vi "_convert_response_to_float_scalar_number.vi"(8 "error in":errorcluster caption="error in (no error)", 10 "Input string":string, 11 "VISA resource name":refnum<visa-resource-name>) -> (0 "error out":errorcluster, 2 "Double out":dbl format="%#_p", 3 "VISA resource name out":refnum<visa-resource-name>)   [LabVIEW 2020, in "Rohde&Schwarz RTx Oscilloscopes.lvlib" / "rsidr_core.lvlib"]
doc: "Queries array of floats that can be returned in ASCII format or in binary format. The array is always returned as the most-universal double array.\n- For <b>ASCII</b> format, the array numbers are decoded as comma-separated values.\n- For <b>Binary Format</b>, the numbers are decoded based on the session parameter <b>Bin Float Number Format</b>, usually float 32-bit (REAL,32), swapped endianess (instruments usually use low endian, LabVIEW uses big endian)."
uses:
  rsidr_core.lvlib
  type_AdditionalFlag_Bits.ctl
  type_Error_Codes.ctl
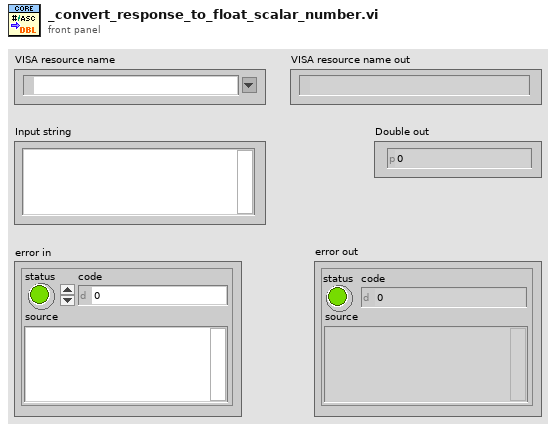
[diagram p1: front panel]
types:
  T1 = typedef "Rohde&Schwarz RTx Oscilloscopes.lvlib/rsidr_core.lvlib/type_AdditionalFlag_Bits.ctl" = enum16{"Send LF after Bin Block", "Junk read with io_clear_buffers.vi", "io_clear_buffers: viClear()", "io_clear_buffers: viFlush()", "<NotUsed1>", "Allow Dbl & Int Bin/Ascii read", "*OPC? in check_instrument_error.vi", "<NotUsed2>", "Smart Enum Matching", "Less Strict RepCaps check", "AssureResponseEndWithLF"}
  T2 = typedef "Rohde&Schwarz RTx Oscilloscopes.lvlib/rsidr_core.lvlib/type_Error_Codes.ctl" = enum16{"No_error", "VISA_err_ResourceNotFound", "VISA_err_Timeout", "VISA_warn_MoreDataAvailable", "RS_err_MissingCallback", "RS_err_InvalidAttribute", "RS_err_InvalidValue", "RS_err_UnknownResource", "RS_err_AlreadyInitialized", "RS_err_InstrumentStatus", "RS_err_BadRepCapName", "RS_err_TypesMismatch", "RS_err_ValueNotSupported", "RS_err_InvalidRngTable", "RS_err_IDqueryFail", "RS_err_UnexpResponse", "VISA_warn_ConfigNotLoaded", "RS_err_AttributeNotReadable", "RS_err_AttributeNotWritable", "RS_err_InstrumentType", "RS_err_InstrumentOption", "VISA_err_InvalidSize", "RS_err_ReliabilityIndicator", "VISA_warn_UnknownStatus", "VISA_warn_TermCharRead", "VISA_err_IO_error", "RS_err_FunctionNotSupported", "VISA_warn_QueueEmpty"}
  T3 = typedef "Rohde&Schwarz RTx Oscilloscopes.lvlib/rsidr_core.lvlib/type_Session_Data.ctl" = cluster{"IDN string":string, "Instrument FW":string, "Instr type":string, "Instr type for err. msg.":string, "Installed Options":string[], "Ignore Error Messages":string, "Logging params":variant, "OPC Timeout":i32, "VISA Timeout":i32, "STB Poll VISA Timeout":i32, "Additional Flags":i32, "Wait Before Read":i32, "Wait Before Write":i32, "Option String Flags":i32, "IO Segment Size":i64, "VISA Access Mode":T4, "Interface Type":T5, "OPC Wait Mode":T6, "Bin Float Number  Format":T7, "Bin Integer Number Format":T8, "Simulate":bool, "VXIcapable":bool, "Duplicate Session":bool, "Add LF to Write":bool, "Logging":bool, "Fast Sweep":bool, "Query Instrument Status":bool, "Check Range":bool, "Check Options":bool, "OPC-sync Attr Writes":bool, "OPC-sync Attr Queries":bool}
  T4 = typedef "Rohde&Schwarz RTx Oscilloscopes.lvlib/rsidr_core.lvlib/type_VisaAccessMode.ctl" = u16
  T5 = typedef "Rohde&Schwarz RTx Oscilloscopes.lvlib/rsidr_core.lvlib/type_InterfaceType.ctl" = enum16{"Unknown", "GPIB", "VXI", "GPIB_VXI", "ASRL", "PXI", "TCPIP", "USB", "SOCKET"}
  T6 = typedef "Rohde&Schwarz RTx Oscilloscopes.lvlib/rsidr_core.lvlib/type_OPC_Wait_Mode.ctl" = enum16{"STBpolling", "STBpollingSlow", "STBpollingSuperSlow", "ServiceRequest", "OPCquery"}
  T7 = typedef "Rohde&Schwarz RTx Oscilloscopes.lvlib/rsidr_core.lvlib/type_Binary_Float_Number_Format.ctl" = enum16{"Float_4_Bytes_Swapped", "Float_4_Bytes", "Double_8_Bytes_Swapped", "Double_8_Bytes"}
  T8 = typedef "Rohde&Schwarz RTx Oscilloscopes.lvlib/rsidr_core.lvlib/type_Binary_Integer_Number_Format.ctl" = enum16{"Int32_4_Bytes_Swapped", "Int32_4 Bytes", "Int16_2_Bytes_Swapped", "Int16_2_Bytes"}
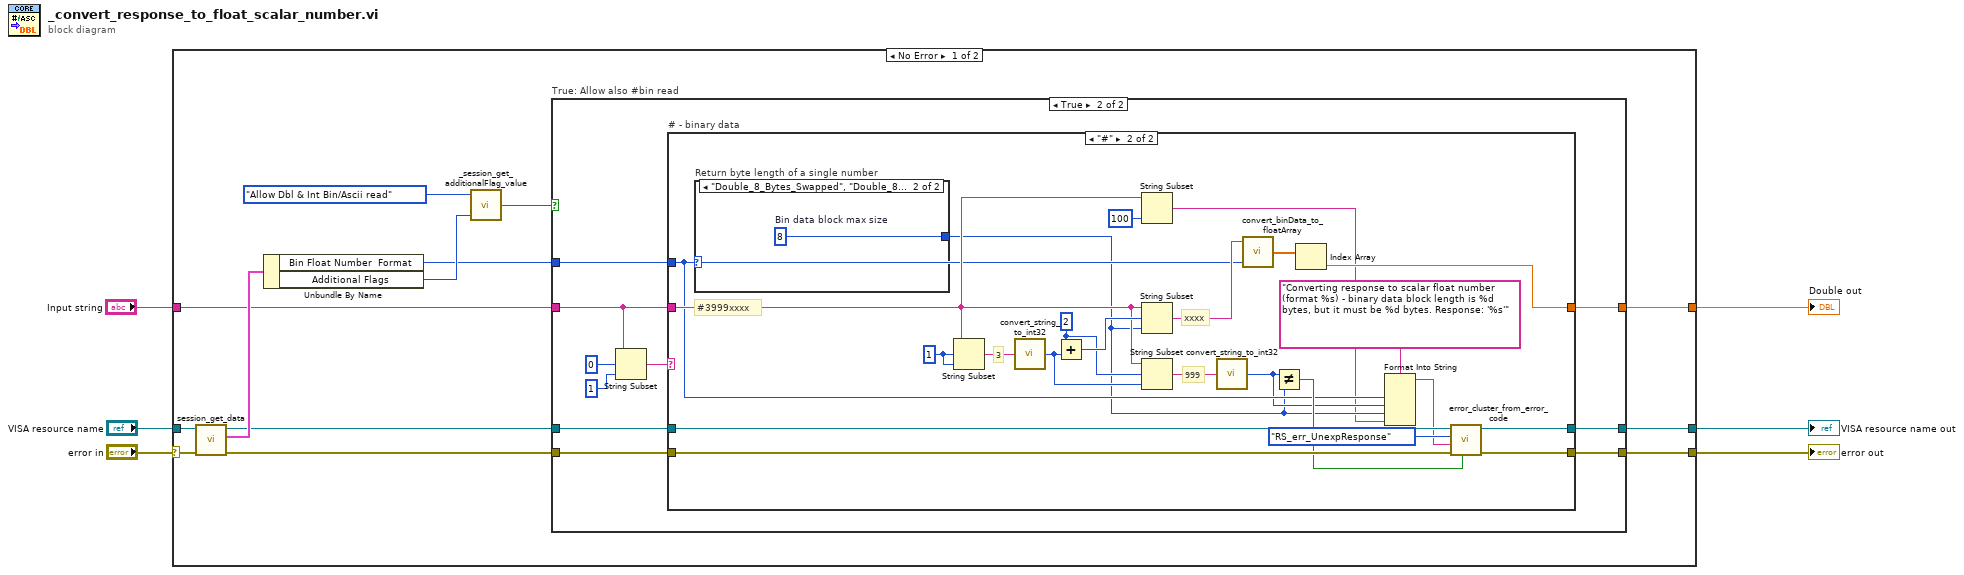
[diagram p0: block diagram]
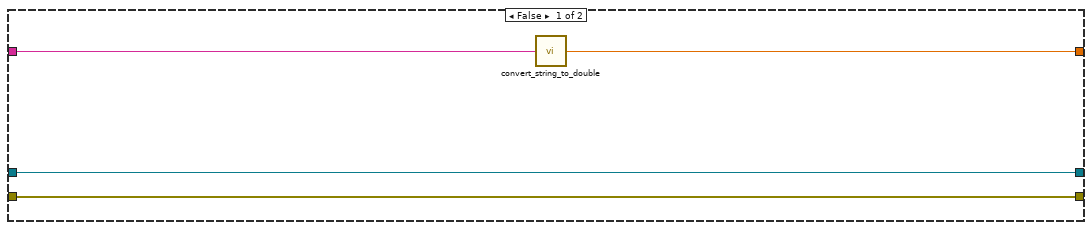
[diagram p2: hidden frame]
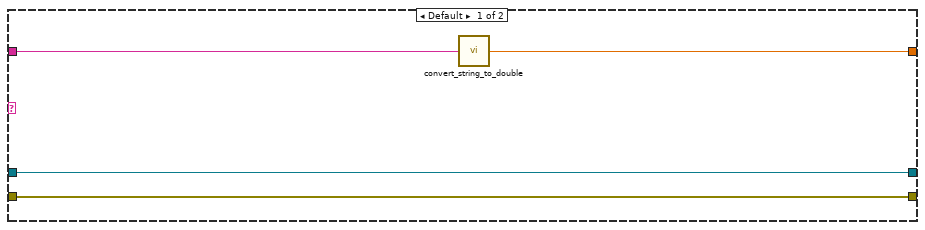
[diagram p3: hidden frame]
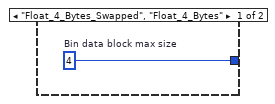
[diagram p4: hidden frame]
diagram:
  n1 = case shown="No Error" "error in" {
    selector: "error in" -> [w19 w64]
    tunnel: [w7 w63] -> w3
    tunnel: [w8 w64] -> w4
    tunnel: "VISA resource name" -> [w18 w63]
    tunnel: [w12 _] -> w1
    tunnel: "Input string" -> [w11 _]
    frame No Error {
      n2 = call "session_get_data.vi"("error in"=w19, "VISA resource name"=w18) -> ("error out"=w10:errorcluster, "Session User Data out"=w17:T3, "VISA resource name out"=w9:refnum<visa-resource-name>)  [unwired: 6 in, 1 out]
      n3 = Unbundle By Name(w17) -> ("Bin Float Number  Format"=w14:T7, "Additional Flags"=w15:i32)
      n4 = call "_session_get_additionalFlag_value.vi"("AdditionalFlags value in"=w15, "AdditionalFlag bit"=type_AdditionalFlag_Bits."Allow Dbl & Int Bin/Ascii read") -> ("AdditionalFlag bit value out"=w13:bool)  [unwired: 3 in]
      n5 = case "True: Allow also #bin read" shown="True" w13 {
        tunnel: w14 -> [_ w25]
        tunnel: [w22 w27] -> w12
        tunnel: w11 -> [w23 w26]
        tunnel: w10 -> [w21 w30]
        tunnel: w9 -> [w20 w31]
        tunnel: [w21 w28] -> w8
        tunnel: [w20 w29] -> w7
        frame False {
          n6 = call "convert_string_to_double.vi"("String in"=w23) -> ("double value out"=w22:dbl)  [unwired: 4 in]
        }
        frame True {
          n7 = String Subset(string=w26, offset (0)=0, length (rest)=1 ("length (rest)")) -> (substring=w24:string)
          n8 = case "# - binary data" shown="\"#\"" w24 {
            tunnel: w26 -> [w37 w43]
            tunnel: w25 -> [_ w41]
            tunnel: [w36 w56] -> w27
            tunnel: w30 -> [w35 w50]
            tunnel: w31 -> [w34 w49]
            tunnel: [w35 w48] -> w28
            tunnel: [w34 w47] -> w29
            frame Default {
              n9 = call "convert_string_to_double.vi"("String in"=w37) -> ("double value out"=w36:dbl)  [unwired: 4 in]
            }
            frame "#" {
              w54 = 2 ("offset (0)")
              w60 = 1 ("offset (0)")
              # "xxxx"
              # "999"
              # "3"
              # "#3999xxxx"
              n10 = case "Return byte length of a single number" shown="\"Double_8_Bytes_Swapped\", \"Double_8_Bytes\"" w41 {
                tunnel: [w61 w62] -> w39
                frame "Float_4_Bytes_Swapped", "Float_4_Bytes" {
                  w61 = 4  # Bin data block max size
                }
                frame "Double_8_Bytes_Swapped", "Double_8_Bytes" {
                  w62 = 8  # Bin data block max size
                }
              }
              n11 = String Subset(string=w43, offset (0)=w60, length (rest)=w60) -> (substring=w59:string)
              n12 = call "convert_string_to_int32.vi"("String in"=w59) -> ("int32 value out"=w53:i32)  [unwired: 4 in]
              n13 = Add(x=w54, y=w53) -> (x+y=w55:i32)
              n14 = String Subset(string=w43, length (rest)=100 ("length (rest)")) -> (substring=w38:string)  [unwired: 1 in]
              n15 = String Subset(string=w43, offset (0)=w55, length (rest)=w39) -> (substring=w58:string)
              n16 = String Subset(string=w43, offset (0)=w54, length (rest)=w53) -> (substring=w52:string)
              n17 = call "convert_string_to_int32.vi"("String in"=w52) -> ("int32 value out"=w40:i32)  [unwired: 4 in]
              n18 = call "convert_binData_to_floatArray.vi"("Bin Float Number Format"=w41, "Bin Data"=w58) -> ("Numbers out"=w57:dbl[])  [unwired: 1 in, 2 out]
              n19 = Not Equal?(x=w40, y=w39) -> (x != y?=w46:bool)
              n20 = Index Array(array=w57) -> (element=w56:dbl)  [unwired: 1 in]
              n21 = Format Into String(format string="Converting response to scalar float number (format %s) - binary data block length is %d bytes, but it must be %d bytes. Response: '%s'", w41, w40, w39, w38) -> (resulting string=w44:string)  [unwired: 2 in, 1 out]
              n22 = call "error_cluster_from_error_code.vi"("Error Creation Enabled (True)"=w46, "error in"=w50, "Error Message (\"\")"=w44, "Error Enum in"=type_Error_Codes."RS_err_UnexpResponse", "VISA resource name"=w49) -> ("error out"=w48:errorcluster, "VISA resource name out"=w47:refnum<visa-resource-name>)  [unwired: 5 in]
            }
          }
        }
      }
    }
    frame Error {
    }
  }
  "error out" <- w4
  "VISA resource name out" <- w3
  "Double out" <- w1
